vi "Receive.vi"(1 "Topic name":string, 2 "MQTT_API in":refnum<class "MQTT_API.lvclass">) -> (0 "Message":string)   [LabVIEW 2019]
uses:
  <vilib>/addons/WireFlow/_WireQueue/MQTT API/MQTT_API.lvclass
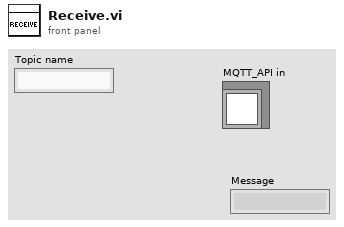
[diagram p1: front panel]
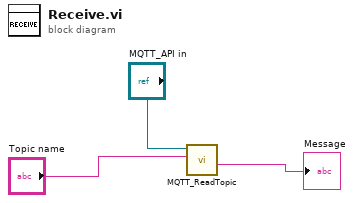
[diagram p0: block diagram]
diagram:
  n1 = call <vilib>:"MQTT_ReadTopic.vi"("Topic name"="Topic name", "MQTT_API in"="MQTT_API in") -> ("Value"=→"Message":string)  [unwired: 5 in, 4 out]
